vi "Save EventLog.vi"(8 "error in (no error)":errorcluster, 11 "EventLog in":refnum<class "EventLog.lvclass">) -> (0 "error out":errorcluster, 3 "EventLog out":refnum<class "EventLog.lvclass">)   [LabVIEW 2019, in "EventLog.lvclass"]
uses:
  EventLog.lvclass
  7b7a7308-cd97-4965-baa9-19cd06179aec.vi
  Events/Events.lvclass
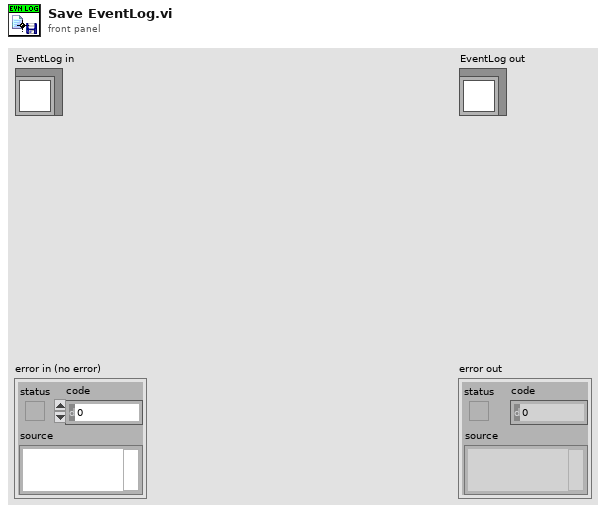
[diagram p1: front panel]
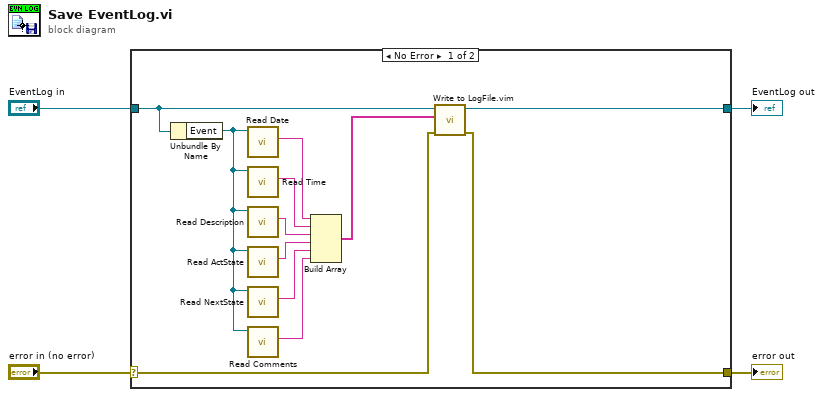
[diagram p0: block diagram]
diagram:
  n1 = case shown="No Error" "error in (no error)" {
    selector: "error in (no error)" -> [w6 w18]
    tunnel: [w5 w18] -> w3
    tunnel: [w15 w17] -> w1
    tunnel: "EventLog in" -> [w16 w17]
    frame No Error {
      n2 = Unbundle By Name(w16) -> ("Event"=w14:refnum<class "Events.lvclass">)
      n3 = call "Read Date.vi"("Events in"=w14) -> ("Date"=w8:string)  [unwired: 8 in, 2 out]
      n4 = call "Read Time.vi"("Events in"=w14) -> ("Time"=w11:string)  [unwired: 8 in, 2 out]
      n5 = call "Read Description.vi"("Events in"=w14) -> ("Description"=w12:string)  [unwired: 8 in, 2 out]
      n6 = call "Read ActState.vi"("Events in"=w14) -> ("ActState"=w13:string)  [unwired: 8 in, 2 out]
      n7 = call "Read NextState.vi"("Events in"=w14) -> ("NexttState"=w10:string)  [unwired: 8 in, 2 out]
      n8 = call "Read Comments.vi"("Events in"=w14) -> ("Comments"=w9:string)  [unwired: 8 in, 2 out]
      n9 = Build Array(w8, w11, w12, w13, w10, w9) -> (w7:string[])
      n10 = call "Write to LogFile.vim"("Error In"=w6, "Data"=w7, "LogClass In"=w16) -> ("Error out"=w5:errorcluster, "LogClass Out"=w15:refnum<class "EventLog.lvclass">)  [unwired: 7 in]
    }
    frame Error {
    }
  }
  "error out" <- w3
  "EventLog out" <- w1
